vi "Incoming Bit.vi"(8 "error in (no error)":errorcluster, 10 "Incoming Bit (Get)":cluster{"Address":u16, "Set/Reset":bool}, 11 "Controller in":refnum<class "Controller.lvclass">) -> (0 "error out":errorcluster, 3 "Controller out":refnum<class "Controller.lvclass">)   [LabVIEW 2022 SP3, in "Controller.lvlib" / "Controller.lvclass"]
uses:
  Controller.lvclass
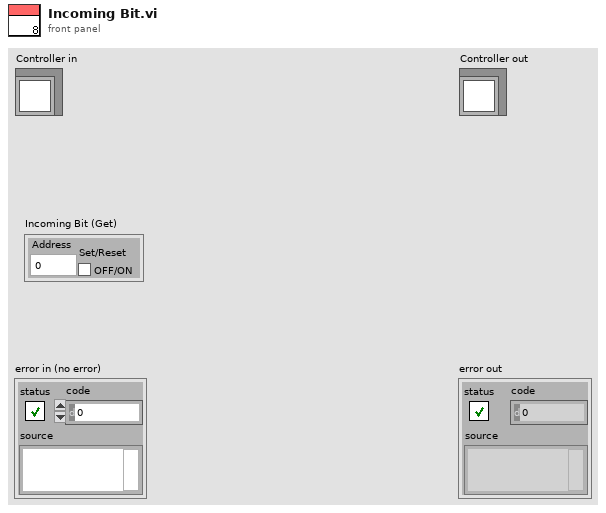
[diagram p1: front panel]
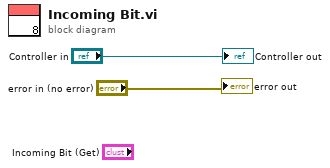
[diagram p0: block diagram]
diagram:
  "error out" <- "error in (no error)"
  "Controller out" <- "Controller in"
